vi "JJMCtarea.vi"() -> ()   [LabVIEW 2013]
panel:
  out "#sobresalientes":dbl
  out "#muybuenos":dbl
  out "#buenos":dbl
  out "#reprobados":dbl
  out "sobresaliente":bool
  out "muy bueno":bool
  out "bueno":bool
  out "reprobados":bool
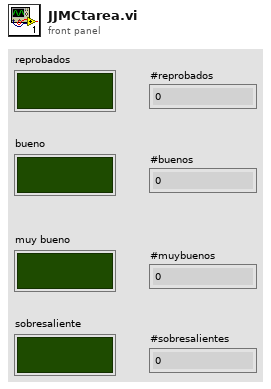
[diagram p1: front panel]
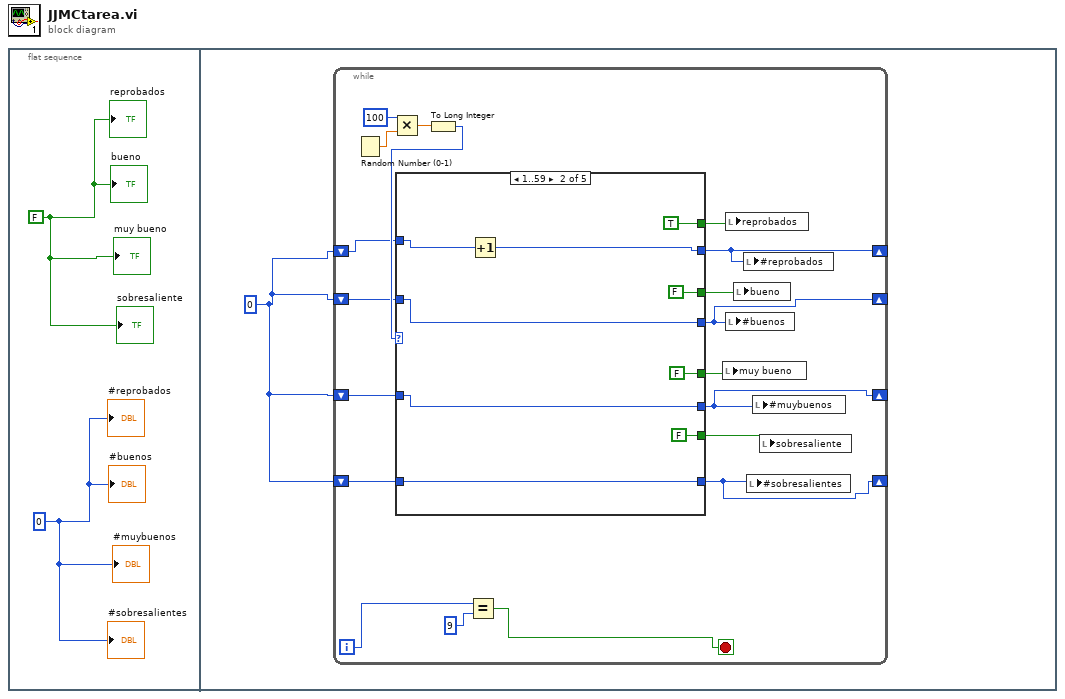
[diagram p0: block diagram]
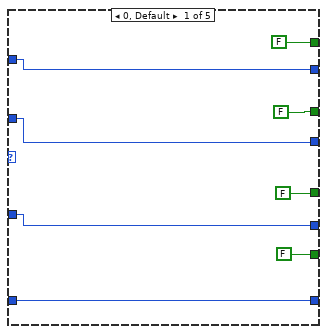
[diagram p2: hidden frame]
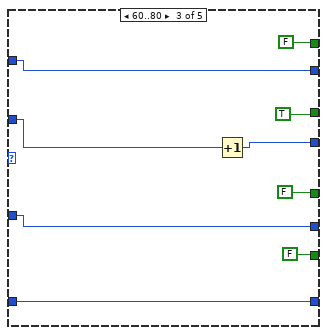
[diagram p3: hidden frame]
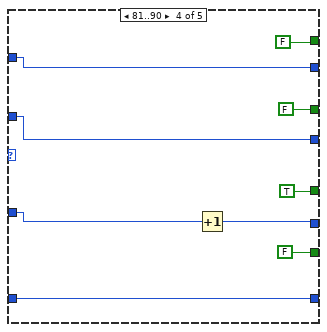
[diagram p4: hidden frame]
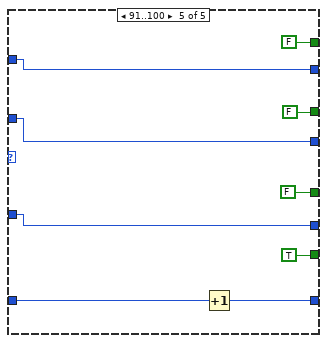
[diagram p5: hidden frame]
diagram:
  n1 = flat-sequence {
    frame #0 {
      w1 = FALSE
      w2 = 0
      "reprobados" <- w1
      "bueno" <- w1
      "muy bueno" <- w1
      "sobresaliente" <- w1
      "#reprobados" <- w2
      "#buenos" <- w2
      "#muybuenos" <- w2
      "#sobresalientes" <- w2
    }
    frame #1 {
      w3 = 0
      n2 = while {
        shift-right: [w4] -> _
        shift-left: w3 -> [w11]
        shift-right: [w5] -> _
        shift-left: w3 -> [w6]
        shift-right: [w7] -> _
        shift-left: w3 -> [w8]
        shift-right: [w9] -> _
        shift-left: w3 -> [w10]
        i -> [w21]
        stop <- w20 stop-if-true
        n3 = Random Number (0-1)() -> (number: 0 to 1=w19:dbl)
        n4 = Multiply(x=100, y=w19) -> (x*y=w17:dbl)
        n5 = To Long Integer(number=w17) -> (32bit integer=w16:i32)
        n6 = case shown="1..59" w16 {
          tunnel: [FALSE TRUE FALSE FALSE FALSE] -> w15
          tunnel: [FALSE FALSE TRUE FALSE FALSE] -> w14
          tunnel: [FALSE FALSE FALSE TRUE FALSE] -> w13
          tunnel: [FALSE FALSE FALSE FALSE TRUE] -> w12
          tunnel: w11 -> [w26 w34 w48 w53 w62]
          tunnel: [w26 w35 w48 w53 w62] -> w4
          tunnel: w10 -> [w25 w31 w40 w51 w59]
          tunnel: [w25 w31 w40 w51 w58] -> w9
          tunnel: w8 -> [w24 w32 w41 w49 w60]
          tunnel: [w24 w32 w41 w50 w60] -> w7
          tunnel: w6 -> [w23 w33 w43 w52 w61]
          tunnel: [w23 w33 w42 w52 w61] -> w5
          frame 0, Default {
          }
          frame 1..59 {
            n7 = Increment(x=w34) -> (x+1=w35:i32)
          }
          frame 60..80 {
            n8 = Increment(x=w43) -> (x+1=w42:i32)
          }
          frame 81..90 {
            n9 = Increment(x=w49) -> (x+1=w50:i32)
          }
          frame 91..100 {
            n10 = Increment(x=w59) -> (x+1=w58:i32)
          }
        }
        n11 = Equal?(x=w21, y=9) -> (x = y?=w20:bool)
        n12 = local write "muy bueno"(w13) -> ()
        n13 = local write "reprobados"(w15) -> ()
        n14 = local write "#buenos"(w5) -> ()
        n15 = local write "bueno"(w14) -> ()
        n16 = local write "#reprobados"(w4) -> ()
        n17 = local write "#sobresalientes"(w9) -> ()
        n18 = local write "#muybuenos"(w7) -> ()
        n19 = local write "sobresaliente"(w12) -> ()
      }
    }
  }
